vi "Handle Payload.vi"(8 "error in (no error)":errorcluster, 10 "Incoming Packets":u8[](array[numeric]) format="%08b", 11 "ControlPacket in":refnum<class "ControlPacket.lvclass">) -> (0 "error out":errorcluster, 1 "Payload Complete?":bool=TRUE, 2 "Remaining Packets":u8[](array[numeric]) format="%08b", 3 "ControlPacket out":refnum<class "ControlPacket.lvclass">)   [LabVIEW 2013, in "MQTT_Control_Packets.lvlib" / "ControlPacket.lvclass"]
uses:
  ControlPacket.lvclass
  ControlPacket.lvclass/ControlPacket.ctl
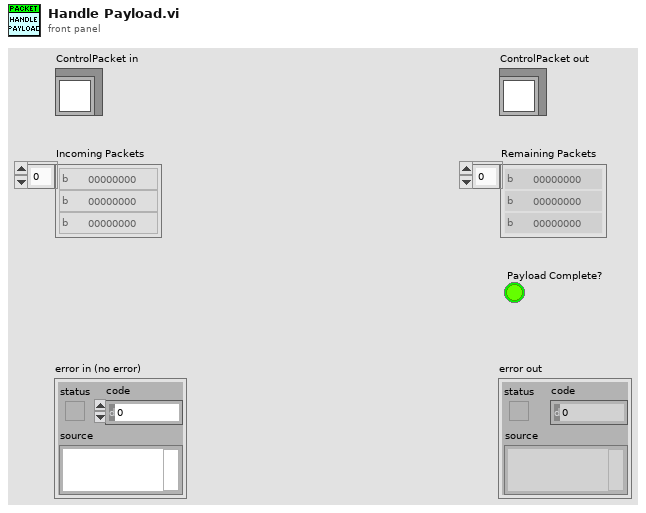
[diagram p1: front panel]
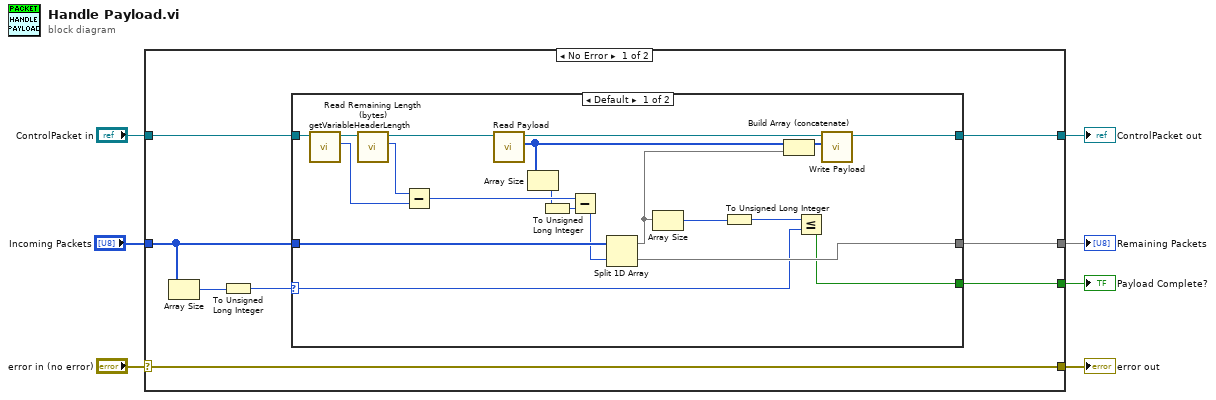
[diagram p0: block diagram]
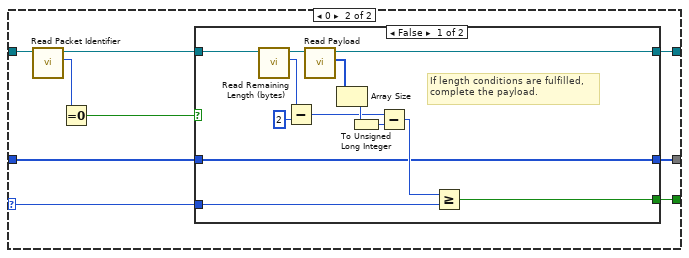
[diagram p2: hidden frame]
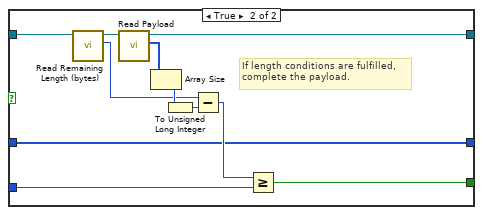
[diagram p3: hidden frame]
diagram:
  n1 = case shown="No Error" "error in (no error)" {
    selector: "error in (no error)" -> [w15 w71]
    tunnel: [w15 w71] -> w6
    tunnel: [w14 w70] -> w4
    tunnel: "ControlPacket in" -> [w8 w70]
    tunnel: "Incoming Packets" -> [w10 w69]
    tunnel: [w13 w69] -> w2
    tunnel: [w12 _] -> w1
    frame No Error {
      n2 = Array Size(array=w10) -> (size(s)=w11:i32)
      n3 = To Unsigned Long Integer(number=w11) -> (unsigned 32bit integer=w9:u32)
      n4 = case shown="Default" w9 {
        selector: w9 -> [w25 w39]
        tunnel: w8 -> [w31 w44]
        tunnel: [w34 w40] -> w14
        tunnel: w10 -> [w33 w37]
        tunnel: [w32 w36] -> w13
        tunnel: [w27 w41] -> w12
        frame Default {
          n5 = call-dynamic "getVariableHeaderLength.vi"("ControlPacket in"=w31) -> ("VariableHeader size"=w29:u32, "ControlPacket out"=w30:refnum<class "ControlPacket.lvclass">)  [unwired: 8 in, 1 out]
          n6 = call "Read Remaining Length (bytes).vi"("ControlPacket in"=w30) -> ("Remaining Length (bytes)"=w28:u32, "ControlPacket out"=w35:refnum<class "ControlPacket.lvclass">)  [unwired: 8 in, 1 out]
          n7 = Subtract(x=w28, y=w29) -> (x-y=w26:u32)
          n8 = call "Read Payload.vi"("ControlPacket in"=w35) -> ("Payload"=w21:u8[], "ControlPacket out"=w24:refnum<class "ControlPacket.lvclass">)  [unwired: 9 in]
          n9 = Array Size(array=w21) -> (size(s)=w23:i32)
          n10 = To Unsigned Long Integer(number=w23) -> (unsigned 32bit integer=w22:u32)
          n11 = Subtract(x=w26, y=w22) -> (x-y=w19:u32)
          n12 = Split 1D Array(array=w33, index=w19) -> (first subarray=w18:u8[], second subarray=w32:u8[])
          n13 = Array Size(array=w18) -> (size(s)=w17:i32)
          n14 = To Unsigned Long Integer(number=w17) -> (unsigned 32bit integer=w16:u32)
          n15 = Build Array (concatenate)(w21, w18) -> (w20:u8[])
          n16 = Less Or Equal?(x=w16, y=w25) -> (x <= y?=w27:bool)
          n17 = call "Write Payload.vi"("Payload"=w20, "ControlPacket in"=w24) -> ("ControlPacket out"=w34:refnum<class "ControlPacket.lvclass">)  [unwired: 9 in]
        }
        frame 0 {
          n18 = call "Read Packet Identifier.vi"("ControlPacket in"=w44) -> ("Packet Identifier"=w42:u16, "ControlPacket out"=w43:refnum<class "ControlPacket.lvclass">)  [unwired: 9 in]
          n19 = Equal To 0?(x=w42) -> (x = 0?=w38:bool)
          n20 = case shown="False" w38 {
            tunnel: w43 -> [w57 w68]
            tunnel: [w49 w62] -> w41
            tunnel: [w48 w61] -> w40
            tunnel: w39 -> [w47 w60]
            tunnel: w37 -> [w45 w58]
            tunnel: [w45 w58] -> w36
            frame False {
              # "If length conditions are fulfilled,\ncomplete the payload."
              n21 = call "Read Remaining Length (bytes).vi"("ControlPacket in"=w57) -> ("Remaining Length (bytes)"=w55:u32, "ControlPacket out"=w56:refnum<class "ControlPacket.lvclass">)  [unwired: 8 in, 1 out]
              n22 = Subtract(x=w55, y=u32 2) -> (x-y=w46:u32)
              n23 = call "Read Payload.vi"("ControlPacket in"=w56) -> ("Payload"=w51:u8[], "ControlPacket out"=w48:refnum<class "ControlPacket.lvclass">)  [unwired: 9 in]
              n24 = Array Size(array=w51) -> (size(s)=w53:i32)
              n25 = To Unsigned Long Integer(number=w53) -> (unsigned 32bit integer=w52:u32)
              n26 = Subtract(x=w46, y=w52) -> (x-y=w50:u32)
              n27 = Greater Or Equal?(x=w50, y=w47) -> (x >= y?=w49:bool)
            }
            frame True {
              # "If length conditions are fulfilled,\ncomplete the payload."
              n28 = call "Read Remaining Length (bytes).vi"("ControlPacket in"=w68) -> ("Remaining Length (bytes)"=w59:u32, "ControlPacket out"=w67:refnum<class "ControlPacket.lvclass">)  [unwired: 8 in, 1 out]
              n29 = call "Read Payload.vi"("ControlPacket in"=w67) -> ("Payload"=w64:u8[], "ControlPacket out"=w61:refnum<class "ControlPacket.lvclass">)  [unwired: 9 in]
              n30 = Array Size(array=w64) -> (size(s)=w66:i32)
              n31 = To Unsigned Long Integer(number=w66) -> (unsigned 32bit integer=w65:u32)
              n32 = Subtract(x=w59, y=w65) -> (x-y=w63:u32)
              n33 = Greater Or Equal?(x=w63, y=w60) -> (x >= y?=w62:bool)
            }
          }
        }
      }
    }
    frame Error {
    }
  }
  "error out" <- w6
  "ControlPacket out" <- w4
  "Remaining Packets" <- w2
  "Payload Complete?" <- w1
